vi "Keyboardshortcuts_171213.vi"   [LabVIEW 2016]
uses:
  Globaltracker.vi
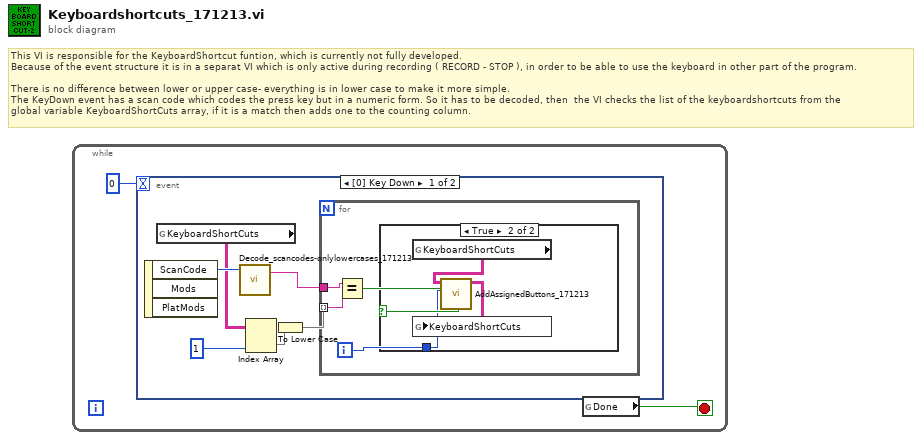
[diagram p0: block diagram]
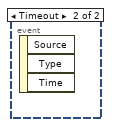
[diagram p3: hidden frame]
diagram:
  # "This VI is responsible for the KeyboardShortcut funtion, which is currently not fully developed.\nBecause of the event structure it is in a separat VI which is only active during recording ( RECORD - STOP ), in order to be able to use the keyboard in other part of the program.\n\nThere is no difference between lower or upper case- everything is in lower case to make it more simple.\nThe KeyDown event has a scan code which codes the press key but in a numeric form. So it has to be decoded, then  the VI checks the list of the keyboardshortcuts from the \nglobal variable KeyboardShortCuts array, if it is a match then adds one to the counting column."
  n1 = while {
    stop <- w1 stop-if-true
    n2 = event shown="[0] Key Down" {
      selector: _ -> [_ _]
      dyn-events: _ -> [_ _]
      timeout: 0 -> [_ _]
      event Key Down {
        n3 = event-data() -> ("ScanCode"=w8:i16)  [unwired: 1 in, 2 out]
        n4 = global read "Globaltracker.vi" "KeyboardShortCuts"() -> (w3:string[][])
        n5 = call "Decode_scancodes-onlylowercases_171213.vi"("ScanCode"=w8) -> ("String"=w6:string)  [unwired: 3 in]
        n6 = Index Array(array=w3, index (col)=1 ("disabled index (col)")) -> (element=w5:string[])  [unwired: 1 in]
        n7 = To Lower Case(string=w5) -> (all lower case string=w4:string[])
        n8 = for {
          tunnel: w6 -> [w12]
          tunnel: w4 -> [w11] mode=indexing
          i -> [w9]
          n9 = Equal?(x=w12, y=w11) -> (x = y?=w10:bool)
          n10 = case shown="True" w10 {
            tunnel: w9 -> [_ w15]
            frame False {
            }
            frame True {
              n11 = global read "Globaltracker.vi" "KeyboardShortCuts"() -> (w14:string[][])
              n12 = call "AddAssignedButtons_171213.vi"("IndexOfTheIncreasedVaule"=w15, "KeyboardShortCutsArray"=w14) -> ("KeyboardShortCutArray"=w13:string[][])  [unwired: 9 in]
              n13 = global write "Globaltracker.vi" "KeyboardShortCuts"(w13) -> ()
            }
          }
        }
      }
      event Timeout {
        n14 = event-data() -> ()  [unwired: 1 in, 3 out]
      }
    }
    n15 = global read "Globaltracker.vi" "Done"() -> (w1:bool)
  }
